vi "ICM Simple Read Program(NoScaling,NoInit).vi"() -> ()   [LabVIEW 2018]
doc: "Test Program.vi\n\nThis is a simple program that uses the ICM to demonstrate its structure.\n\nInstrument Communication Module Version 1.0\nDecember, 2017 Original Code Consulting David Thomson\n www.originalcode.com"
uses:
  Query/Query.lvclass/Query.ctl
  Query/Read Cycle Time (ms).vi
  Parser/Parser.lvclass
  Query/Query.lvclass
  Bus/Bus.lvclass
panel:
  in  "stop":bool
  out "Enabled Channels":string[](array[string])
  out "Data Values":dbl[](array[numeric])
  out "String Read":string
  out "error out":errorcluster
  out "Config File":path
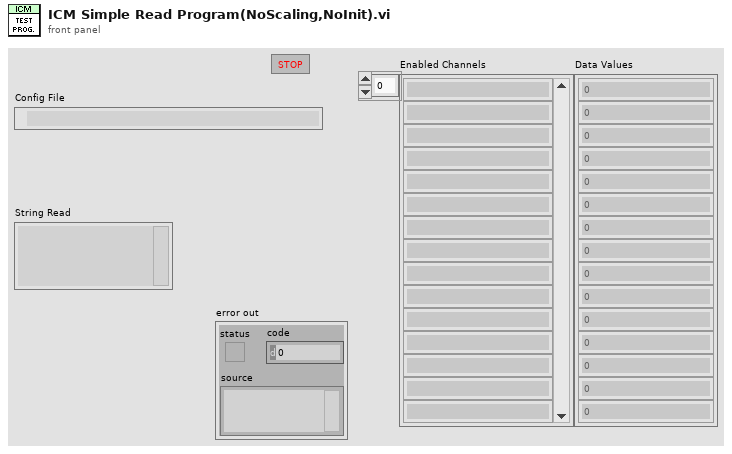
[diagram p1: front panel]
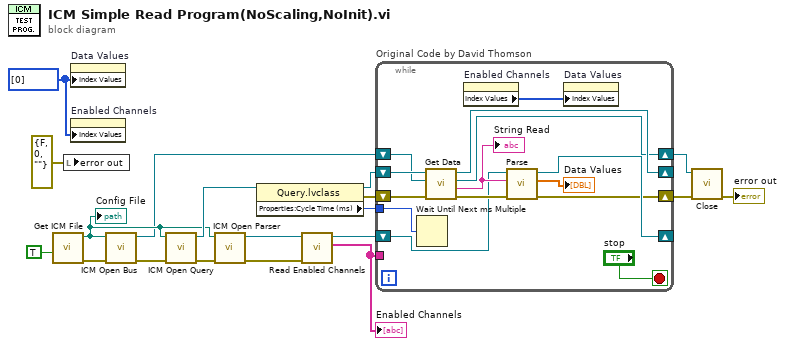
[diagram p0: block diagram]
diagram:
  w3 = u32[] [0] ("Index Values")
  n1 = call "Get ICM File.vi"("Re-Init?"=TRUE) -> ("error out"=w12:errorcluster, "ICM File"=w4:path)  [unwired: 9 in]
  "Config File" <- w4
  n2 = local write "error out"(errorcluster {"status"=FALSE, "code"=0, "source"=""} ("error out")) -> ()
  n3 = property on="Data Values" class="Arr (strict)"("Index Values"=w3) -> ()  [unwired: 2 in, 2 out]
  n4 = property on="Enabled Channels" class="Arr (strict)"("Index Values"=w3) -> ()  [unwired: 2 in, 2 out]
  n5 = call "ICM Open Bus.vi"("error in (no error)"=w12, "ICM File In"=w4) -> ("error out"=w2:errorcluster, "Bus out"=w1:refnum<class "Bus.lvclass">)  [unwired: 8 in]
  n6 = call "ICM Open Query.vi"("error in (no error)"=w2, "ICM File In"=w4) -> ("error out"=w13:errorcluster, "Query out"=w10:refnum<class "Query.lvclass">)  [unwired: 8 in]
  n7 = call "ICM Open Parser.vi"("error in (no error)"=w13, "ICM File In"=w4) -> ("error out"=w14:errorcluster, "Parser out"=w15:refnum<class "Parser.lvclass">)  [unwired: 8 in]
  n8 = property class="Query.lvclass"(reference=w10) -> (reference out=w9:refnum<class "Query.lvclass">, error out=w7:errorcluster, "Properties:Cycle Time (ms)"=w8:u32)  [unwired: 1 in]
  n9 = call-dynamic "Read Enabled Channels.vi"("error in (no error)"=w14, "Parser in"=w15) -> ("Enabled Channels"=w11:string[], "Parser out"=w5:refnum<class "Parser.lvclass">)  [unwired: 7 in, 1 out]
  "Enabled Channels" <- w11
  n10 = while "Original Code by David Thomson" {
    shift-right: [w20] -> w17
    shift-left: w7 -> [w31]
    tunnel: w8 -> [w29]
    tunnel: w11 -> [_]
    shift-right: [w21] -> w18
    shift-left: w1 -> [w28]
    shift-right: [w25] -> _
    shift-left: w5 -> [w26]
    shift-right: [w24] -> _
    shift-left: w9 -> [w32]
    stop <- "stop" stop-if-true
    n11 = Wait Until Next ms Multiple(millisecond multiple=w29) -> ()  [unwired: 1 out]
    n12 = call-dynamic "Get Data.vi"("error in (no error)"=w31, "Bus In"=w28, "Query in"=w32) -> ("error out"=w30:errorcluster, "String Read"=w33:string, "Bus Out"=w21:refnum<class "Bus.lvclass">, "Query out"=w24:refnum<class "Query.lvclass">)  [unwired: 5 in]
    "String Read" <- w33
    n13 = property on="Enabled Channels" class="Arr (strict)"() -> ("Index Values"=w23:u32[])  [unwired: 2 in, 2 out]
    n14 = call-dynamic "Parse.vi"("error in (no error)"=w30, "Data String"=w33, "Parser in"=w26) -> ("error out"=w20:errorcluster, "Data Values"=→"Data Values":dbl[], "Parser out"=w25:refnum<class "Parser.lvclass">)  [unwired: 6 in]
    n15 = property on="Data Values" class="Arr (strict)"("Index Values"=w23) -> ()  [unwired: 2 in, 2 out]
  }
  n16 = call-dynamic "Close.vi"("error in (no error)"=w17, "Bus in"=w18) -> ("error out"=→"error out":errorcluster)  [unwired: 8 in, 1 out]
